vi "Non Actor Test of 6501.vi"() -> ()   [LabVIEW 2016, in "Generic Data Acquisition.lvlib" / "National Instrument USB-6501.lvlib" / "National Instrument USB-6501.lvclass"]
uses:
  National Instrument USB-6501.lvclass
  <vilib>/DAQmx/write.llb/DAQmx Write (Digital Bool 1Line 1Point).vi
  <vilib>/DAQmx/create/channels.llb/DAQmx Create Channel (DO-Digital Output).vi
  <vilib>/DAQmx/miscellaneous.llb/DAQmx Fill In Error Info.vi
panel:
  out "DAQmx Task Name":refnum<k21>
  in  "Port":i8=2
  in  "data":bool
  out "Classic DAQmx Physical Channel":tag
  in  "Line":i8
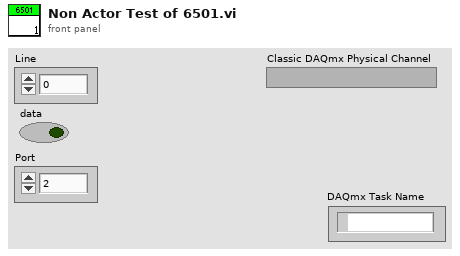
[diagram p1: front panel]
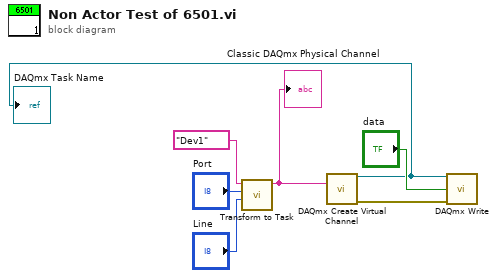
[diagram p0: block diagram]
diagram:
  n1 = call "Transform to Task.vi"("Line"="Line", "Port"="Port", "DAQmx Device Name"=tag "Dev1") -> ("Classic DAQmx Physical Channel"=w4:tag)  [unwired: 8 in]
  "Classic DAQmx Physical Channel" <- w4
  n2 = call-poly <vilib>:"DAQmx Create Virtual Channel.vi"("lines"=w4) -> ("task out"=w1:refnum<k21>, "error out"=w3:errorcluster)  [unwired: 13 in]
  "DAQmx Task Name" <- w1
  n3 = call-poly <vilib>:"DAQmx Write.vi"("task/channels in"=w1, "data"="data", "error in"=w3) -> ()  [unwired: 10 in, 3 out]
